vi "Send.vi"(9 "Priority?":bool, 10 "Msg Strategy":refnum<class "Msg Strategy.lvclass">, 11 "Msg Type Strategy in":refnum<class "Msg Type Strategy.lvclass">) -> (0 "error out":errorcluster)   [LabVIEW 2021, in "jettl.lvlib" / "Msg Type Strategy.lvlib" / "Msg Type Strategy.lvclass"]
uses:
  Msg Type Strategy.lvclass
  Msg Strategy/Msg Strategy.lvclass
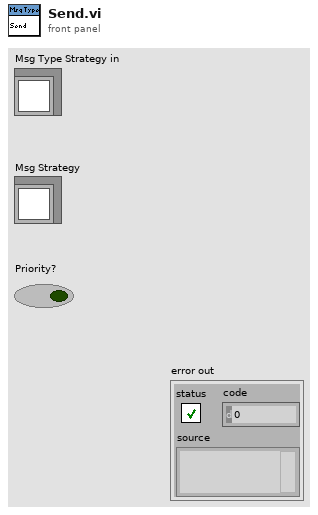
[diagram p1: front panel]
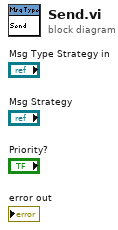
[diagram p0: block diagram]
diagram:
